vi "Launch Connection Factory.vi"(8 "error in (no error)":errorcluster, 11 "PersistantConnectionHandler in":refnum<class "PersistantConnectionHandler.lvclass">) -> (0 "error out":errorcluster, 3 "PersistantConnectionHandler out":refnum<class "PersistantConnectionHandler.lvclass">)   [LabVIEW 2020, in "PersitantConnectionHandler.lvlib" / "PersistantConnectionHandler.lvclass"]
uses:
  <vilib>/gpm_packages/@cs/Network-interface/Source/PersistantConnectionHandler/PersistantConnectionHandler/PersistantConnectionHandler.lvclass
  C:/Program Files/National Instruments/LabVIEW 2020/vi.lib/gpm_packages/@cs/Network-interface/Source/Logged Actor/LoggedActor.lvclass
  <vilib>/gpm_packages/@cs/event-logger/Source/Composed Log/Types/Log Level.ctl
  <vilib>/gpm_packages/@cs/Network-interface/Source/Logged Actor/LoggedActor.lvclass/LoggedActor.ctl
  <vilib>/gpm_packages/@cs/event-logger/Source/Composed Log/LoggerReference/LoggerReference.lvclass/LoggerReference.ctl
  <vilib>/gpm_packages/@cs/Network-interface/Source/PersistantConnectionHandler/PersistantConnectionHandler/PersistantConnectionHandler.lvclass/PersistantConnectionHandler.ctl
  <vilib>/gpm_packages/@cs/event-logger/Source/Composed Log/LoggerReference/Log Event.vi
  <vilib>/gpm_packages/@cs/event-logger/Source/Composed Log/LoggerReference/Log.vi
  <vilib>/gpm_packages/@cs/event-logger/Source/Composed Log/LoggerReference/Get Valid Event Time.vi
  <vilib>/gpm_packages/@cs/event-logger/Source/Composed Log/LoggerReference/Remove Stale Logs.vi
  <vilib>/gpm_packages/@cs/Network-interface/Source/Connection Factory Session/ConnectionFactorySession/ConnectionFactorySession.lvclass
  <vilib>/gpm_packages/@cs/Network-interface/Source/Logged Actor/LoggedActor.lvclass
  <vilib>/gpm_packages/@cs/event-logger/Source/Composed Log/Composed Log.lvlib
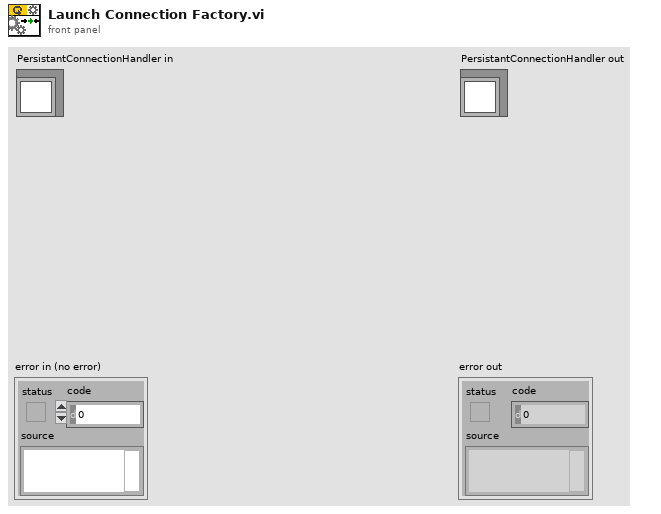
[diagram p1: front panel]
types:
  T1 = typedef "Composed Log.lvlib/Log Level.ctl" = enum16{"Debug", "Info", "Warning", "Error", "Critical"}
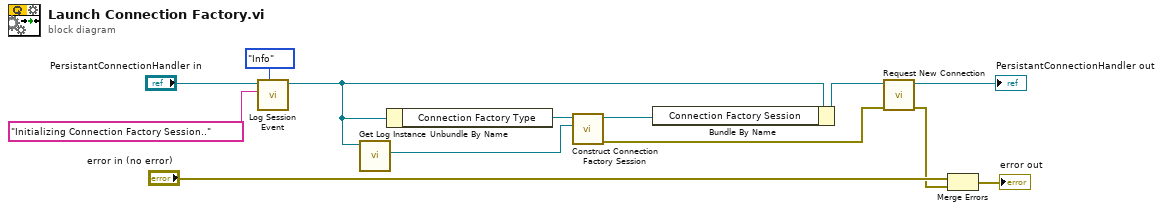
[diagram p0: block diagram]
diagram:
  n1 = call <vilib>:"Log Session Event.vi"("Event Level"=Log_Level."Info", "Event Data"="Initializing Connection Factory Session..", "SessionActor in"="PersistantConnectionHandler in") -> ("SessionActor out"=w2:refnum<class "PersistantConnectionHandler.lvclass">)  [unwired: 7 in, 1 out]
  n2 = call <vilib>:"Get Log Instance.vi"("LoggedActor in"=w2) -> ("Log Instance"=w1:refnum<class "LoggerReference.lvclass">)  [unwired: 8 in, 2 out]
  n3 = Unbundle By Name(w2) -> ("Connection Factory Type"=w13:refnum<class "IConnectionFactory.lvclass">)
  n4 = call <vilib>:"Construct Connection Factory Session.vi"("Log Instance"=w1, "Connection Factory Type"=w13) -> ("error out"=w7:errorcluster, "Connection Factory Session"=w6:refnum<data-value>)  [unwired: 8 in]
  n5 = Bundle By Name(cluster=w2, "Connection Factory Session"=w6) -> (w9:refnum<class "PersistantConnectionHandler.lvclass">)
  n6 = call <vilib>:"Request New Connection.vi"("error in (no error)"=w7, "PersistantConnectionHandler in"=w9) -> ("error out"=w5:errorcluster, "PersistantConnectionHandler out"=→"PersistantConnectionHandler out":refnum<class "PersistantConnectionHandler.lvclass">)  [unwired: 8 in]
  n7 = Merge Errors("error in (no error)", w5) -> (→"error out":errorcluster)
